vi "Suma de ventas.vi"(8 "error in (no error)":errorcluster, 11 "Input cluster":T1) -> (0 "error out":errorcluster, 1 "Array":string[][](array[string]))   [LabVIEW 2020]
panel:
  out "concatenated string":string
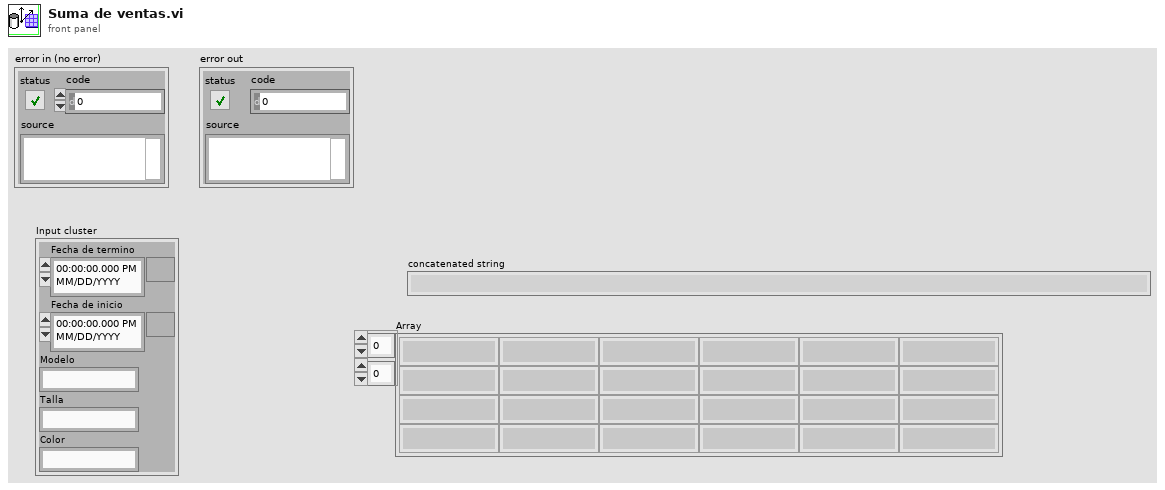
[diagram p1: front panel]
types:
  T1 = cluster{"Fecha de termino":timestamp, "Fecha de inicio":timestamp, "Modelo":string, "Talla":string, "Color":string}
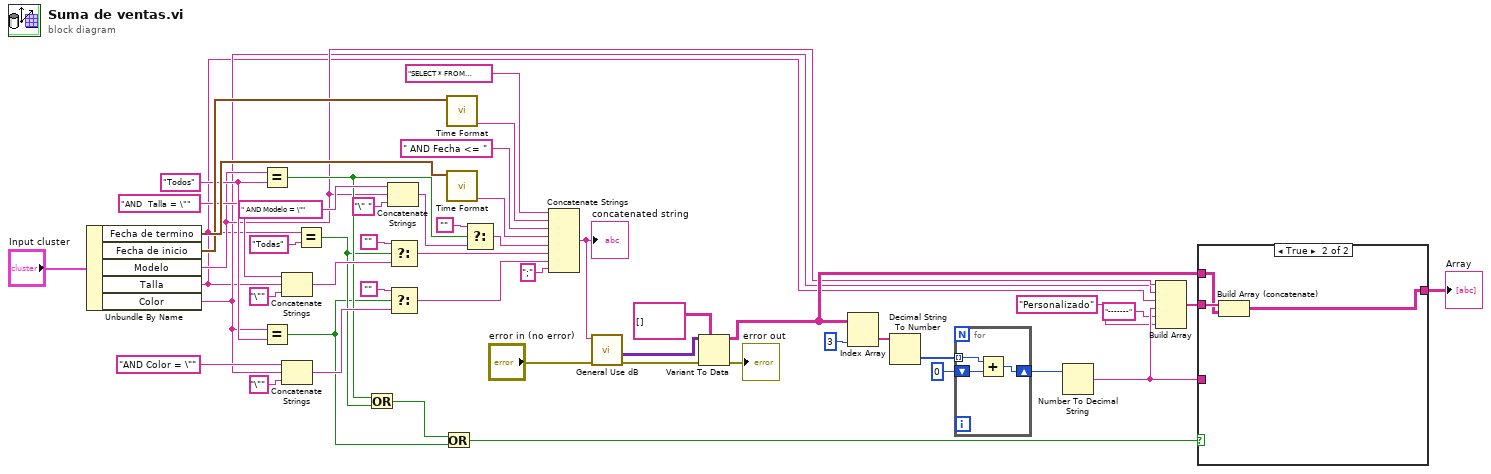
[diagram p0: block diagram]
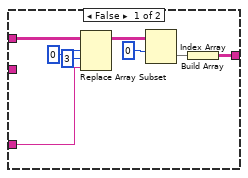
[diagram p2: hidden frame]
diagram:
  w47 = "Todos" ("y")
  n1 = Unbundle By Name("Input cluster") -> ("Fecha de termino"=w49:timestamp, "Fecha de inicio"=w48:timestamp, "Modelo"=w10:string, "Talla"=w8:string, "Color"=w9:string)
  n2 = Equal?(x=w10, y=w47) -> (x = y?=w21:bool)
  n3 = Equal?(x=w9, y=w47) -> (x = y?=w18:bool)
  n4 = Concatenate Strings("AND  Talla = \"" ("string"), w8, "\"" ("string")) -> (w30:string)
  n5 = Concatenate Strings("AND Color = \"" ("string"), w9, "\"" ("string")) -> (w37:string)
  n6 = Equal?(x=w8, y="Todas") -> (x = y?=w20:bool)
  n7 = Or(x=w21, y=w20) -> (x .or. y?=w19:bool)
  n8 = Concatenate Strings(" AND Modelo = \"" ("f"), w10, "\" " ("string")) -> (w39:string)
  n9 = Select(t="", s=w20, f=w30) -> (s? t:f=w31:string)
  n10 = Select(t="", s=w18, f=w37) -> (s? t:f=w29:string)
  n11 = Or(x=w19, y=w18) -> (x .or. y?=w17:bool)
  n12 = call "Time Format.vi"("time stamp"=w48) -> ("concatenated string"=w2:string)  [unwired: 10 in]
  n13 = call "Time Format.vi"("time stamp"=w49) -> ("concatenated string"=w1:string)  [unwired: 10 in]
  n14 = Select(t="", s=w21, f=w39) -> (s? t:f=w42:string)
  n15 = Concatenate Strings("SELECT * FROM Ventas Where Fecha >=  ", w2, " AND Fecha <= " ("string"), w1, w42, w31, w29, ";" ("string")) -> (w27:string)
  "concatenated string" <- w27
  n16 = call "General Use dB.vi"("error in (no error)"="error in (no error)", "Query"=w27) -> ("error out"=w23:errorcluster, "Return Data"=w24:variant[][])  [unwired: 8 in]
  n17 = Variant To Data(error in=w23, type=string[][] [], Variant=w24) -> (data=w11:string[][], error out=→"error out":errorcluster)
  n18 = Index Array(array=w11, index (col)=3 ("disabled index (col)")) -> (element=w14:string[])  [unwired: 1 in]
  n19 = Decimal String To Number(string=w14) -> (number=w15:i32[])  [unwired: 2 in, 1 out]
  n20 = for {
    tunnel: w15 -> [w53] mode=indexing
    shift-right: [w52] -> w16
    shift-left: 0 -> [w51]
    n21 = Add(x=w53, y=w51) -> (x+y=w52:i32)
  }
  n22 = Number To Decimal String(number=w16) -> (decimal integer string=w7:string)  [unwired: 1 in]
  n23 = Build Array(w10, w9, w8, w7, "-------", "Personalizado" ("element")) -> (w4:string[])
  n24 = case shown="True" w17 {
    tunnel: w11 -> [w59 w63]
    tunnel: w7 -> [w55 _]
    tunnel: [w57 w62] -> w3
    tunnel: w4 -> [_ w64]
    frame False {
      n25 = Replace Array Subset(array=w59, new element=w55, index (row)=0, index (col)=3 ("disabled index (col)")) -> (w61:string[][])
      n26 = Index Array(array=w61, index (row)=0) -> (element=w58:string[])  [unwired: 1 in]
      n27 = Build Array(w58) -> (w57:string[][])
    }
    frame True {
      n28 = Build Array (concatenate)(w64, w63) -> (w62:string[][])
    }
  }
  "Array" <- w3
